vi "Initialize.vi"(8 "error in (no error)":errorcluster, 11 "JSON RPC in":refnum<class "JSON RPC.lvclass">) -> (0 "error out":errorcluster, 3 "JSON RPC out":refnum<class "JSON RPC.lvclass">)   [LabVIEW 2016, in "JSON RPC.lvclass"]
uses:
  JSON RPC.lvclass
  JSON RPC.lvclass/JSON RPC.ctl
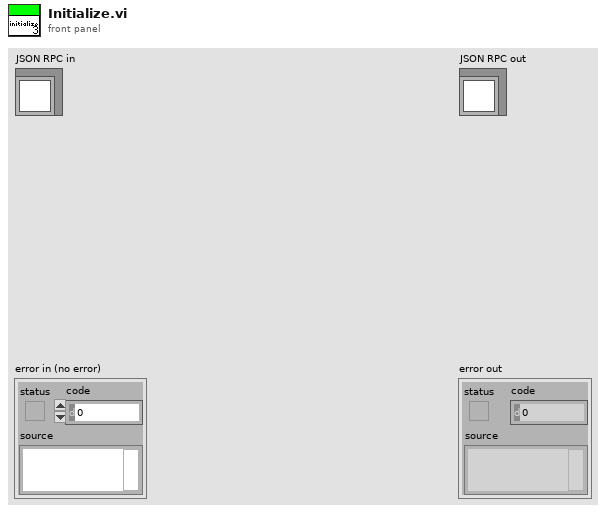
[diagram p1: front panel]
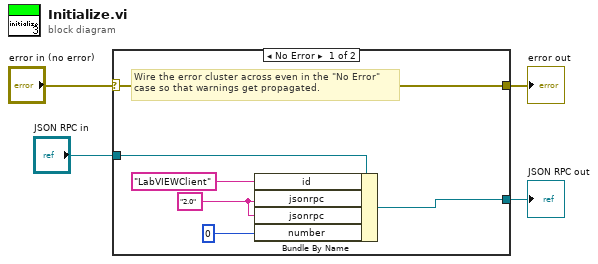
[diagram p0: block diagram]
diagram:
  n1 = case shown="No Error" "error in (no error)" {
    selector: "error in (no error)" -> [w10 w12]
    tunnel: [w10 w12] -> w3
    tunnel: [w8 w11] -> w1
    tunnel: "JSON RPC in" -> [w9 w11]
    frame No Error {
      w5 = "2.0" ("jsonrpc")
      # "Wire the error cluster across even in the \"No Error\"\ncase so that warnings get propagated."
      n2 = Bundle By Name(cluster=w9, "id"="LabVIEWClient", "jsonrpc"=w5, "jsonrpc"=w5, "number"=0) -> (w8:refnum<class "JSON RPC.lvclass">)
    }
    frame Error {
    }
  }
  "error out" <- w3
  "JSON RPC out" <- w1
